vi "CMD_ALERT.vi"(6 "Gantry in":refnum<class "Gantry.lvclass">, 8 "error in (no error)":errorcluster, 10 "Arguments":string[](array[string]), 11 "gScript Interpreter in":refnum<class "gScript Interpreter.lvclass">) -> (0 "error out":errorcluster, 3 "gScript Interpreter out":refnum<class "gScript Interpreter.lvclass">, 4 "Gantry out":refnum<class "Gantry.lvclass">)   [LabVIEW 2024, in "gScript Interpreter.lvclass"]
uses:
  gScript Interpreter.lvclass
  gScript Interpreter.lvclass/gScript Interpreter.ctl
  Shared Components/Gantry Class/Gantry.lvclass
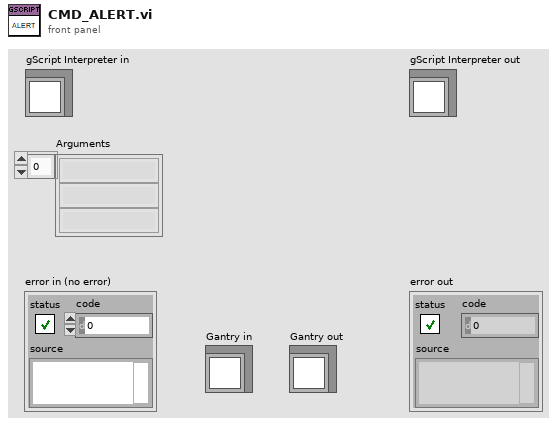
[diagram p1: front panel]
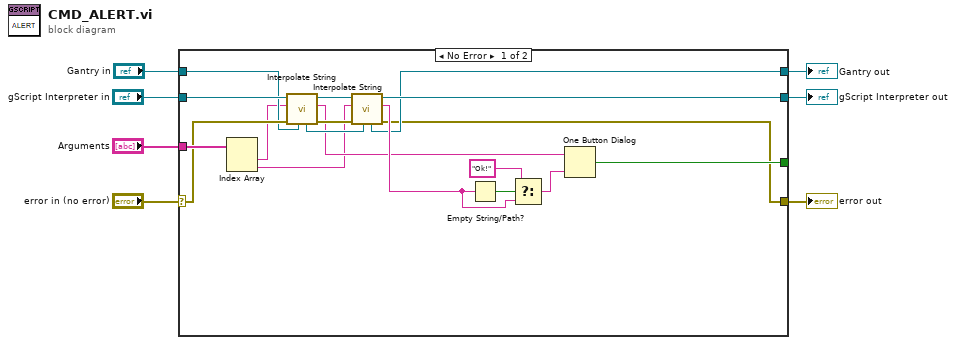
[diagram p0: block diagram]
diagram:
  n1 = case shown="No Error" "error in (no error)" {
    selector: "error in (no error)" -> [w20 w28]
    tunnel: [w8 w28] -> w6
    tunnel: [w13 w27] -> w4
    tunnel: "gScript Interpreter in" -> [w22 w27]
    tunnel: "Arguments" -> [w25 _]
    tunnel: "Gantry in" -> [w17 w26]
    tunnel: [w12 w26] -> w1
    tunnel: [w9 _] -> _
    frame No Error {
      n2 = Index Array(array=w25) -> (element #1=w11:string, element #2=w10:string)  [unwired: 2 in]
      n3 = call-dynamic "Interpolate String.vi"("Gantry in"=w17, "error in (no error)"=w20, "Input String"=w11, "gScript Interpreter in"=w22) -> ("error out"=w19:errorcluster, "Output String"=w15:string, "gScript Interpreter out"=w21:refnum<class "gScript Interpreter.lvclass">, "Gantry out"=w16:refnum<class "Gantry.lvclass">)  [unwired: 4 in]
      n4 = call-dynamic "Interpolate String.vi"("Gantry in"=w16, "error in (no error)"=w19, "Input String"=w10, "gScript Interpreter in"=w21) -> ("error out"=w8:errorcluster, "Output String"=w18:string, "gScript Interpreter out"=w13:refnum<class "gScript Interpreter.lvclass">, "Gantry out"=w12:refnum<class "Gantry.lvclass">)  [unwired: 4 in]
      n5 = Empty String/Path?(string/path=w18) -> (empty?=w24:bool)
      n6 = Select(t="Ok!", s=w24, f=w18) -> (s? t:f=w14:string)
      n7 = One Button Dialog(message=w15, button name ("OK")=w14) -> (true=w9:bool)
    }
    frame Error {
    }
  }
  "error out" <- w6
  "gScript Interpreter out" <- w4
  "Gantry out" <- w1
